vi "RecoverdBaseData_Core.vi"() -> ()   [LabVIEW 2011]
uses:
  <vilib>/addons/database/Connection.llb/Conn ObjectReference.ctl
  <vilib>/addons/database/Connection.llb/DB Tools Open Connec (String).vi
  <vilib>/addons/database/Connection.llb/Conn Execute.vi
  <vilib>/addons/database/Recordset.llb/Rec Destroy - Connection.vi
  <vilib>/addons/database/NI_Database_API.lvlib
panel:
  in  "database name":string
  in  "userID":string="codis_med_wrt"
  out "dup path":path
  in  "Folder":string="C:\\CoDiS\\"
  out "SQL":string
  out "error out":errorcluster
  out "Connection \nreference OUT":T1
  in  "Connection reference IN":T1
  in  "error IN":errorcluster
  in  "Table":string="tvector"
  # "( Must finish with \"\\\" )"
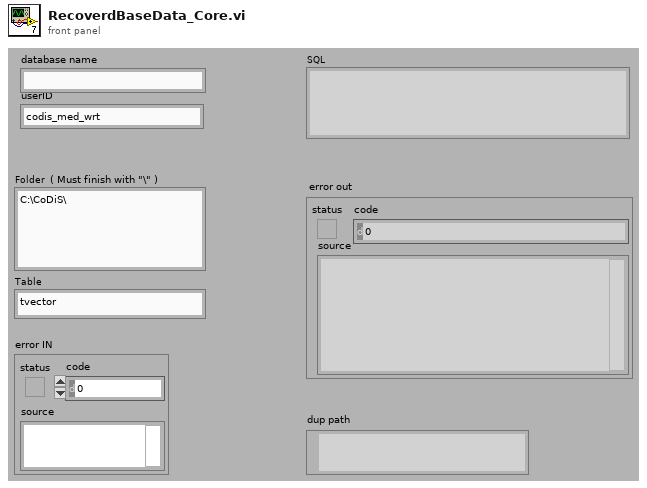
[diagram p1: front panel]
types:
  T1 = typedef "NI_Database_API.lvlib/Conn ObjectReference.ctl" = refnum<k1>
  T2 = typedef "NI_Database_API.lvlib/Rec ObjectReference.ctl" = refnum<k1>
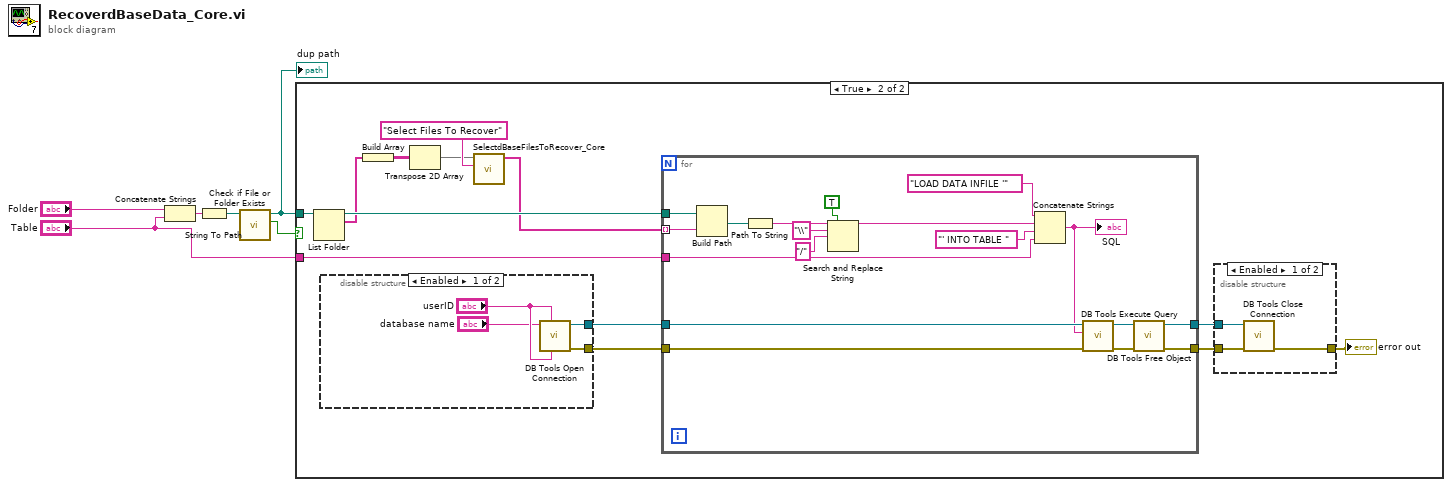
[diagram p0: block diagram]
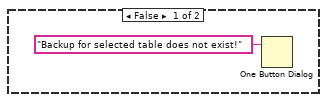
[diagram p2: hidden frame]
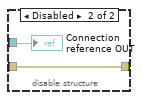
[diagram p3: hidden frame]
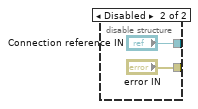
[diagram p4: hidden frame]
diagram:
  n1 = Concatenate Strings("Folder", "Table") -> (w5:string)
  n2 = String To Path(string=w5) -> (path=w4:path)
  n3 = call <vilib>:"Check if File or Folder Exists.vi"("path"=w4) -> ("file or folder exists?"=w2:bool, "dup path"=w3:path)  [unwired: 8 in, 1 out]
  "dup path" <- w3
  n4 = case shown="True" w2 {
    tunnel: w3 -> [_ w20]
    tunnel: "Table" -> [_ w18]
    frame False {
      n5 = One Button Dialog(message="Backup for selected table does not exist!") -> ()  [unwired: 1 in, 1 out]
    }
    frame True {
      n6 = List Folder(path=w20) -> (path out=w19:path, filenames=w12:string[])  [unwired: 3 in, 2 out]
      n7 = disable-structure shown="Enabled" {
        disable-tunnel: [w27 "Connection reference IN"] -> w17
        disable-tunnel: [w26 "error IN"] -> w16
        frame Enabled {
          n8 = call-poly <vilib>:"DB Tools Open Connection.vi"("password"="userID", "userID"="userID", "connection information"="database name") -> ("error out"=w26:errorcluster, "connection reference"=w27:T1)  [unwired: 5 in]
        }
        frame Disabled {
        }
      }
      n9 = Build Array(w12) -> (w9:string[][])
      n10 = Transpose 2D Array(2D array=w9) -> (transposed array=w8:string[][])
      n11 = call "SelectdBaseFilesToRecover_Core.vi"("Description"="Select Files To Recover", "Files To Recover"=w8) -> ("Selected Files"=w10:string[])  [unwired: 7 in]
      n12 = for {
        tunnel: w19 -> [w49]
        tunnel: w10 -> [w48] mode=indexing
        tunnel: w18 -> [w39]
        tunnel: w17 -> [w38]
        tunnel: w16 -> [w37]
        tunnel: [w32] -> w15
        tunnel: [w33] -> w14
        n13 = Build Path(base path=w49, name or relative path=w48) -> (appended path=w47:path)
        n14 = Path To String(path=w47) -> (string=w46:string)
        n15 = Search and Replace String(replace all?=TRUE ("replace all? (F)"), input string=w46, search string="\\", replace string="/" ("replace string (\"\")")) -> (result string=w41:string)  [unwired: 4 in, 3 out]
        n16 = Concatenate Strings("LOAD DATA INFILE '" ("search string"), w41, "' INTO TABLE " ("string"), w39) -> (w36:string)
        "SQL" <- w36
        n17 = call-poly <vilib>:"DB Tools Execute Query.vi"("error in (no error)"=w37, "SQL query"=w36, "connection reference"=w38) -> ("error out"=w34:errorcluster, "recordset reference"=w35:T2)  [unwired: 5 in]
        n18 = call-poly <vilib>:"DB Tools Free Object.vi"("error in (no error)"=w34, "recordset reference"=w35) -> ("error out"=w33:errorcluster, "connection reference"=w32:T1)  [unwired: 8 in]
      }
      n19 = disable-structure shown="Enabled" {
        disable-tunnel: w15 -> [w23 w24]
        disable-tunnel: w14 -> [w22 w25]
        disable-tunnel: [w21 w25] -> w13
        frame Enabled {
          n20 = call <vilib>:"DB Tools Close Connection.vi"("error in (no error)"=w22, "connection reference"=w23) -> ("error out"=w21:errorcluster)  [unwired: 5 in]
        }
        frame Disabled {
          "Connection \nreference OUT" <- w24
        }
      }
      "error out" <- w13
    }
  }
